vi "Reference Names Global.vi"() -> ()   [LabVIEW 2017]
panel:
  in  "Gamepad":string
  in  "Right Joystick - Left & Right":string
  in  "Left Joystick - Forward & Reverse":string
  out "Climb Motor":string="Climb Motor"
  out "Gear IR":string="Gear IR"
  out "Left Drive Slave 2":string="Left Drive Slave 2"
  out "Left Drive Slave 1":string="Left Drive Slave 1"
  out "Right Drive Slave 2":string="Right Drive Slave 2"
  out "Right Drive Slave 1":string="Right Drive Slave 1"
  out "Gear Chute Door":string="Gear Chute Door"
  out "Pigeon IMU":string="Pigeon IMU"
  out "Shooter IR Sensor":string="Shooter IR Sensor"
  out "LED Pattern Boolean 3":string="LED Pattern Boolean 3"
  out "Shooter Slave":string="Shooter Slave"
  out "Climbing Servo":string="Climbing Servo"
  out "Copilot Controller":string="Copilot Controller"
  out "LED Pattern Boolean 2":string="LED Pattern Boolean 2"
  out "LED Pattern Boolean 1":string="LED Pattern Boolean 1"
  out "LED Pattern Boolean 0":string="LED Pattern Boolean 0"
  out "Gear Intake Actuator":string="Gear Intake Actuator"
  out "Gear Release Actuator":string="Gear Paddle Actuator"
  out "Right Lift Drive Gear Shifter":string="Right Lift Drive Gear Shifter"
  out "Left Lift Drive Gear Shifter":string="Left Lift Drive Gear Shifter"
  out "Drive Speed Gear Shifter":string="Drive Speed Gear Shifter"
  out "Pilot Controller":string="Pilot Controller"
  out "Ball Intake Master":string="Ball Intake Master"
  out "Ball Conveyor":string="Ball Conveyor"
  out "Shooter Master":string="Shooter Master"
  out "Right Drive Master":string="Right Drive Master"
  out "Left Drive Master":string="Left Drive Master"
  in  "Left and Right Motors":string
  # "Joysticks"
  # "Motors"
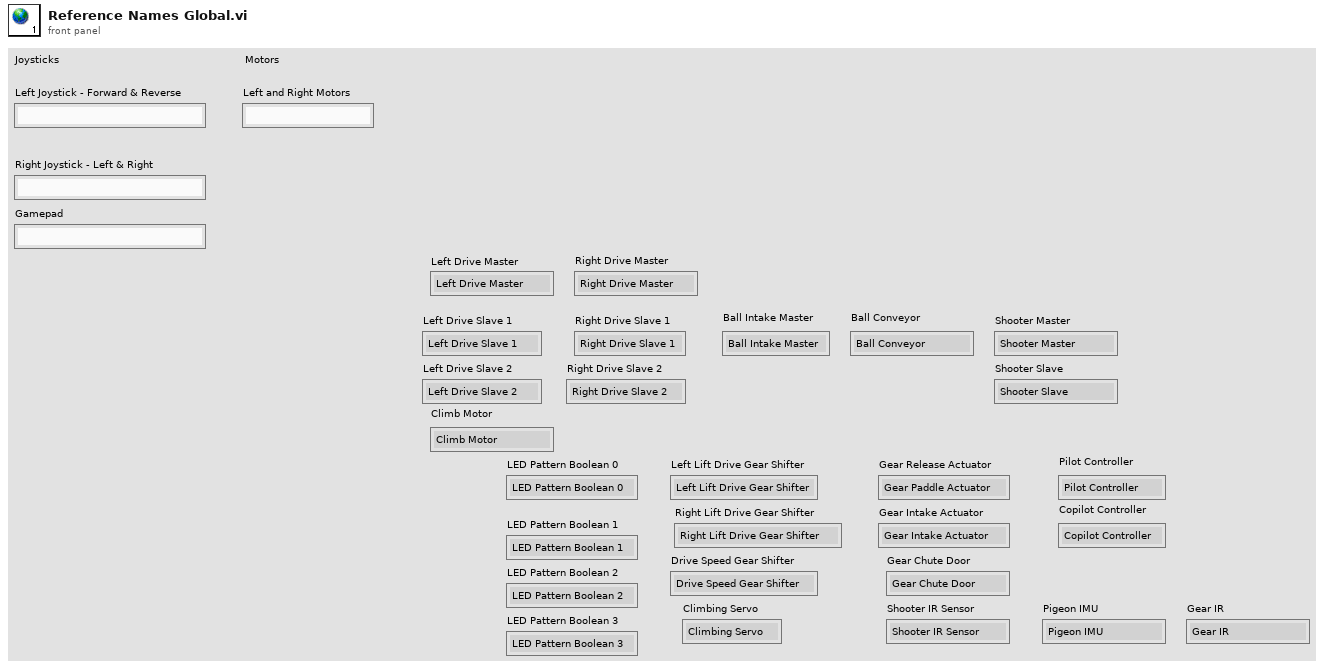
[diagram p1: front panel]
diagram:
